vi "Main.vi"() -> ()   [LabVIEW 2017]
doc: "Le programme Main est l'IHM principal du programme MonoSelector. Il controle le sélecteur d'onde de la manipe \"FastFlim\". Il acquit le spectre du laser et permet de positioner le sélecteur ainsi que de choisir la bande passante des ondes lumineuse."
uses:
  Devices/Laser/PulsePickerValues.ctl
  Lib IHM Control/MHL Data.ctl
  Lib IHM Control/MHL UI Data.ctl
  Lib IHM Control/MHL UI Ref.ctl
  Lib IHM Control/Front Panel Status.ctl
  Fonction de transfert/Convertion.ctl
  Lib QMH/MessageQueues.lvlib
  Lib Notifier/Notifier.lvlib
  Lib IHM Control/IHM Control.lvlib
  Lib Log/Logging.lvlib
panel:
  in  "Pulse Picker Set":T1 items=["80"=80, "40"=40, "20"=20, "10"=10, ""=0]
  out "Laser Connection":bool
  in  "LaserON":bool
  out "Power":dbl
  in  "LaserOFF":bool
  out "Pulse Picker":dbl
  in  "Power Set (%)":u8 max=100
  in  "Abort":bool
  in  "Integration (ms)":i32=100
  in  "Stop":bool
  in  "View":bool
  in  "Dlambda +":bool
  in  "Step (mm)":dbl=0.1
  out "lambda":dbl
  in  "Dlambda -":bool
  out "Position (mm)":dbl
  in  "Target (nm)":dbl=480.0
  out "Mono Selector Status":string
  out "Spectrer":cluster{"X":dbl, "Y":dbl}[](graph)
  # "Spectrometer"
  # "Lambda Select"
  # "Laser"
  # "Slite Wide"
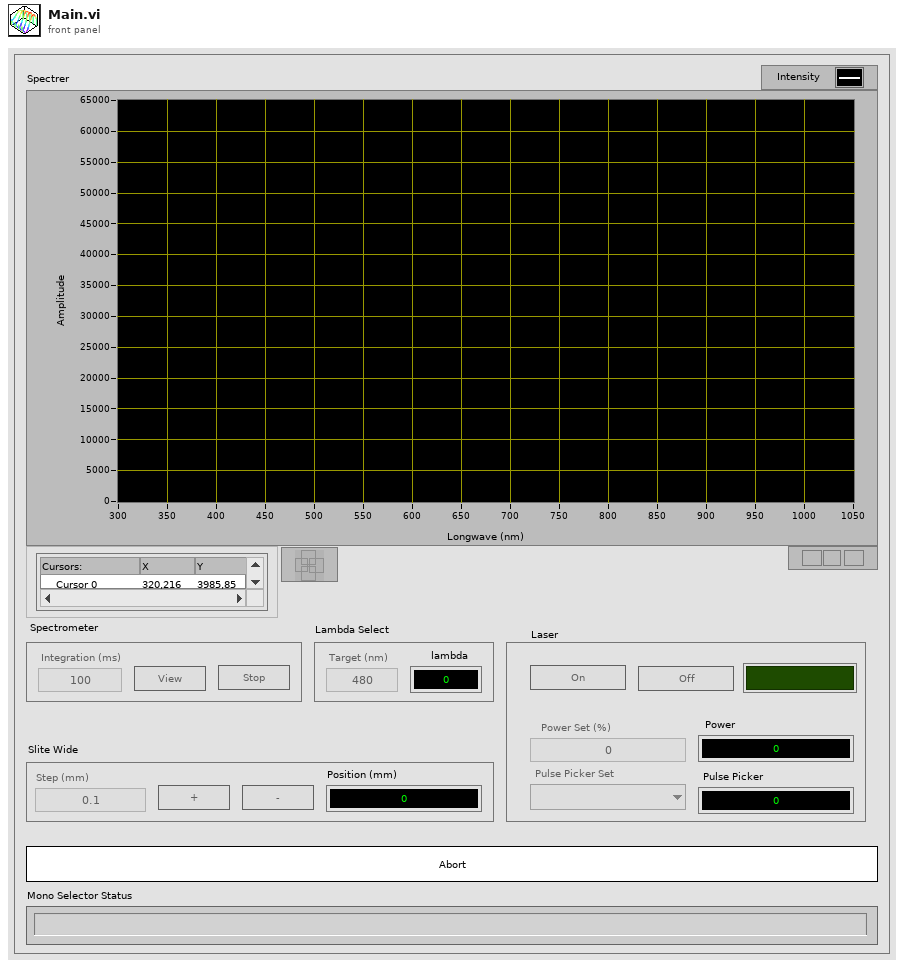
[diagram p1: front panel]
types:
  T1 = typedef "PulsePickerValues.ctl" = u16
  T2 = typedef "MHL Data.ctl" = cluster{"IHM Data":T3, "MHL ref":T4, "Front Panel status":T5}
  T3 = typedef "MHL UI Data.ctl" = cluster{"Integration":i32, "Target Lambda":dbl, "Lambda":dbl, "Step":dbl, "Status Mono":string, "Specter":cluster{"X":dbl, "Y":dbl}[], "Delta Lambda":dbl, "Laser":bool, "Laser Power":dbl, "Pulse Picker Rep. Rate":dbl}
  T4 = typedef "IHM Control.lvlib/MHL UI Ref.ctl" = cluster{"Dlambda-":refnum<vi>, "Abort":refnum<vi>, "Dlambda +":refnum<vi>, "Stop":refnum<vi>, "View":refnum<vi>, "Integration":refnum<vi>, "Target ":refnum<vi>, "Step ":refnum<vi>, "Laser Connection":refnum<vi>, "Power":refnum<vi>, "LaserON":refnum<vi>, "LaserOFF":refnum<vi>, "Pulse Picker Set":refnum<vi>}
  T5 = typedef "IHM Control.lvlib/Front Panel Status.ctl" = enum16{"Initialisation", "Enable Slit", "Enable Positionner", "Enable Spectrometer", "Enable Laser", "Disable Slit", "Disable Positionner", "Disable Spectrometer", "Disable Laser"}
  T6 = typedef "MessageQueues.lvlib/AllMessageQueue Cluster.ctl" = cluster{"MHL":refnum<queue>, "Manager":refnum<queue>, "Recipe":refnum<queue>, "Slit":refnum<queue>, "Positioner":refnum<queue>, "Laser":refnum<queue>, "Spectrometer":refnum<queue>, "Slit Controller":refnum<queue>, "Positioner Controller":refnum<queue>, "Spectrometer Controller":refnum<queue>, "Laser Controller":refnum<queue>}
  T7 = typedef "Notifier.lvlib/Notifier.ctl" = cluster{"Slit Handshake":refnum<notifier>, "Slit Ctrl Exit":refnum<notifier>, "Slit Exit":refnum<notifier>, "Pos. Hanshake":refnum<notifier>, "Pos. Ctrl Exit":refnum<notifier>, "Pos. Exit":refnum<notifier>, "Spectro. Hanshake":refnum<notifier>, "Spectro. Ctrl Exit":refnum<notifier>, "Spectro. Exit":refnum<notifier>, "Laser Handshake":refnum<notifier>, "Laser Ctrl Exit":refnum<notifier>, "Laser Exit":refnum<notifier>}
  T8 = typedef "Convertion.ctl" = enum16{"LongW to Pos.", "Pos. To longW"}
  T9 = enum32{"Invalid", "Standard", "Closed", "Hidden", "Minimized", "Maximized"}
  T10 = enum16{"open", "replace", "create", "open or create", "replace or create", "replace or create with confirmation"}
  T11 = cluster{"état":bool, "code":i32, "source":string}
  T12 = enum32{"invalid app kind", "Development System", "Run Time System", "Student Edition", "Embedded LabVIEW", "Evaluation", "Custom"}
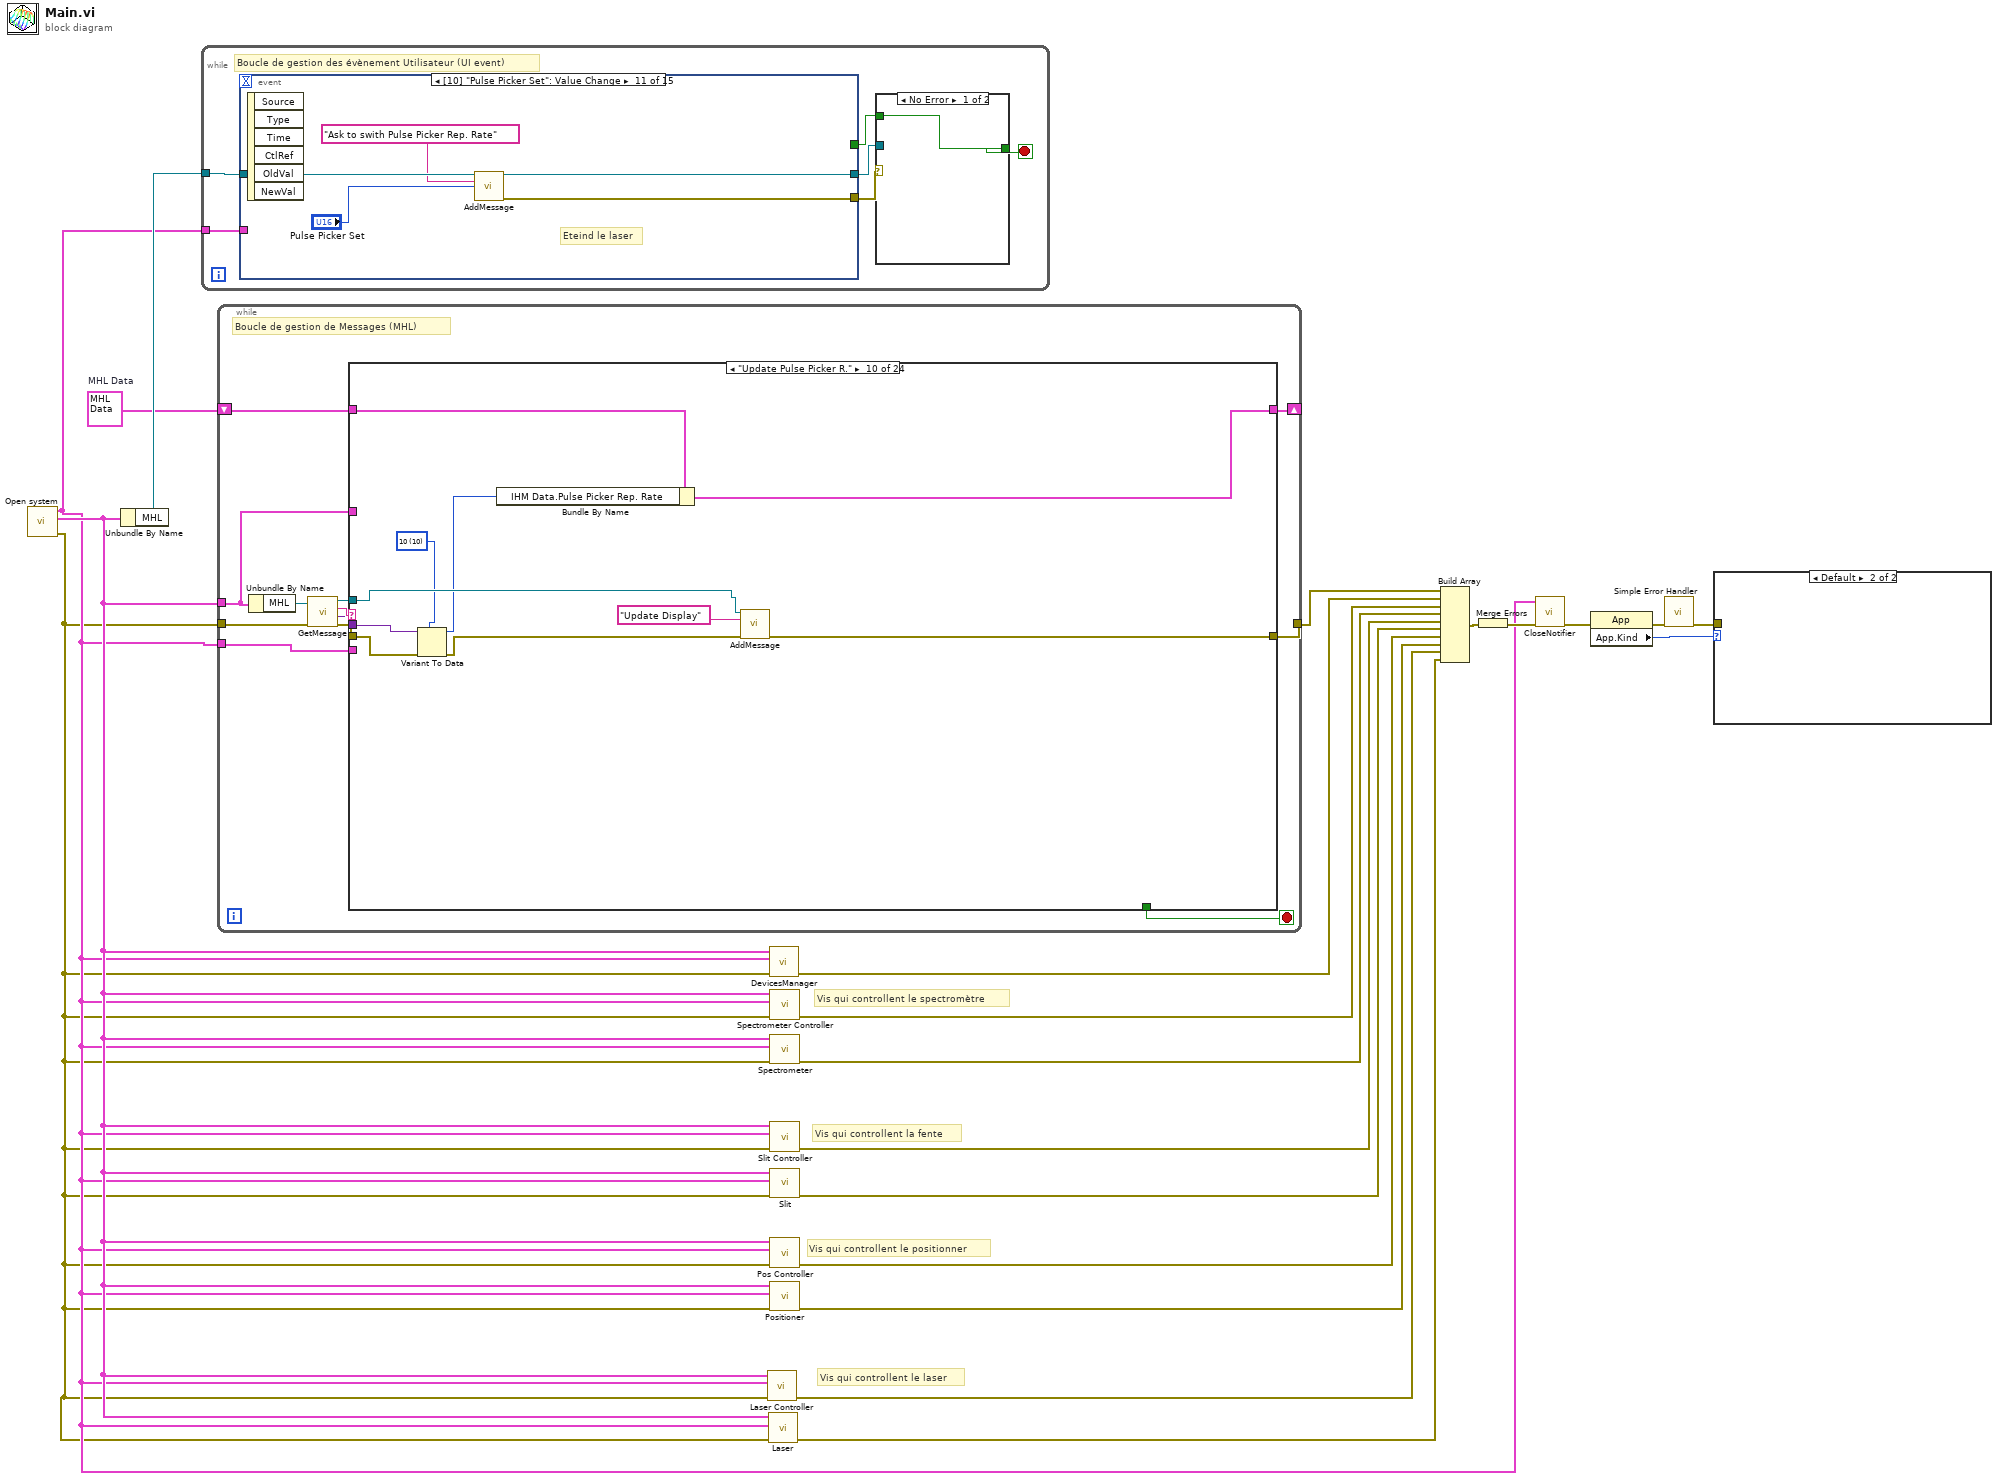
[diagram p0: block diagram]
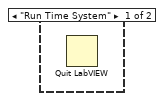
[diagram p2: hidden frame]
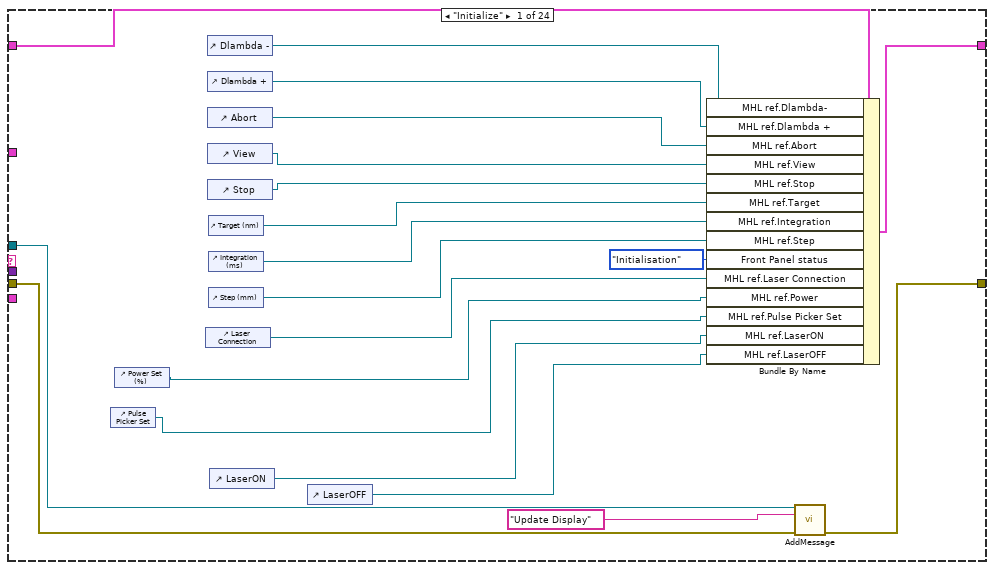
[diagram p3: hidden frame]
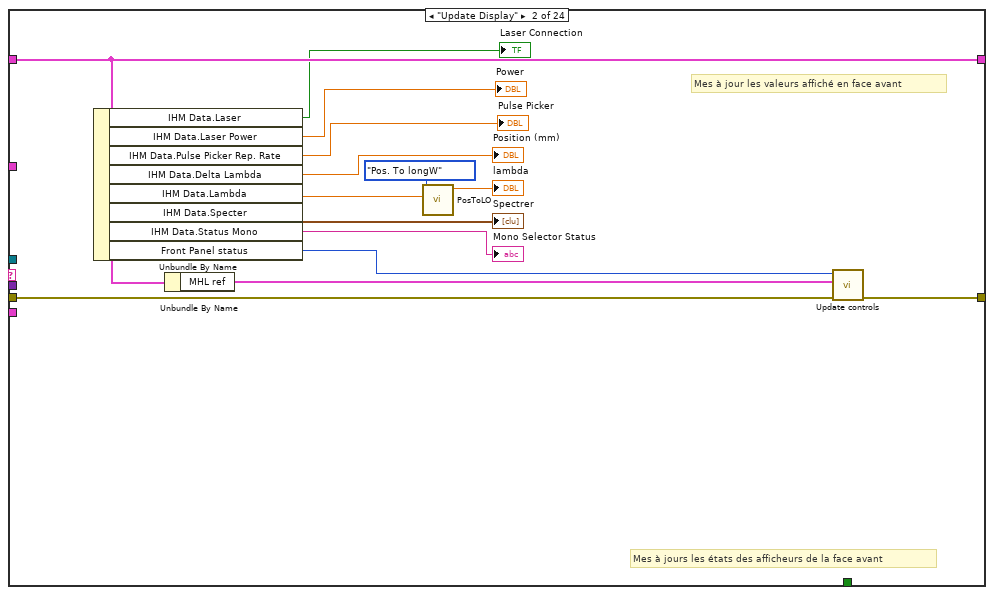
[diagram p4: hidden frame]
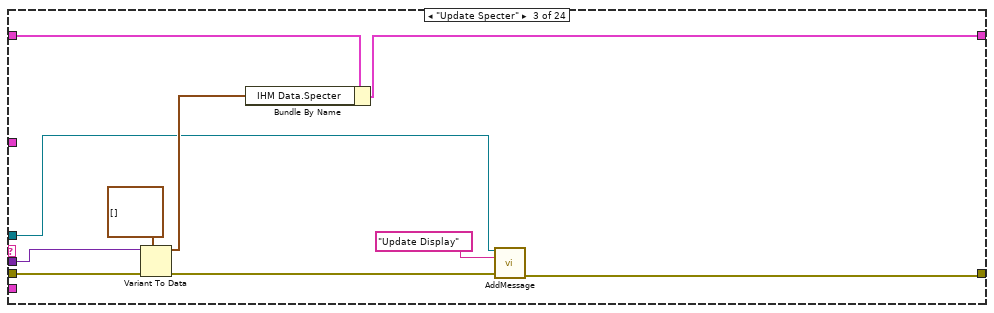
[diagram p5: hidden frame]
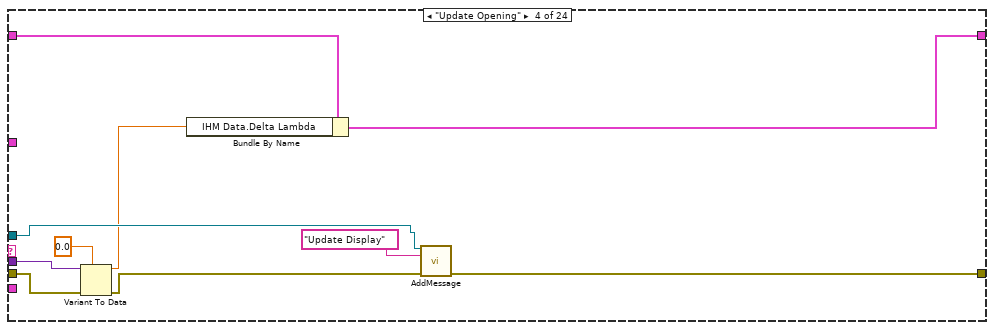
[diagram p6: hidden frame]
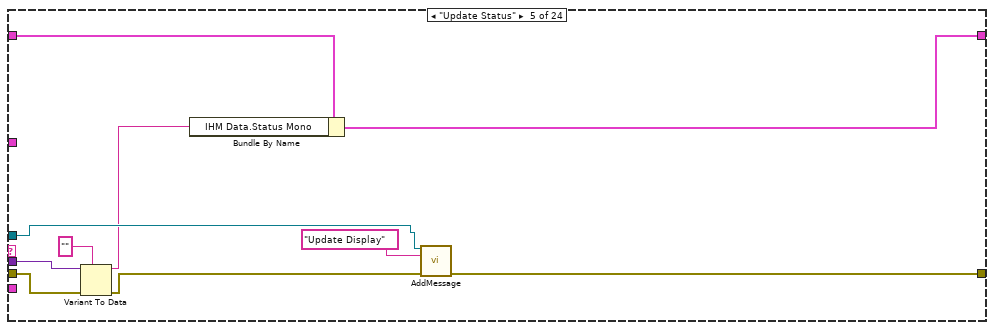
[diagram p7: hidden frame]
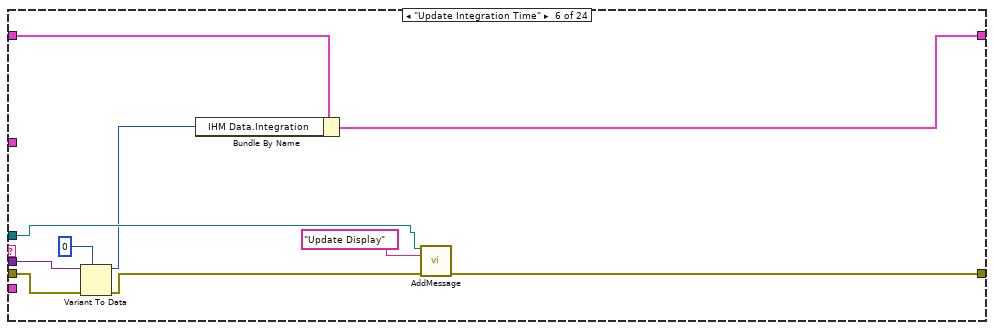
[diagram p8: hidden frame]
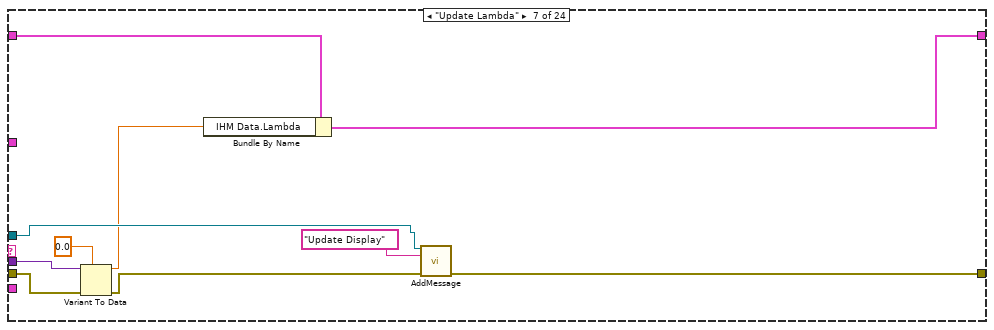
[diagram p9: hidden frame]
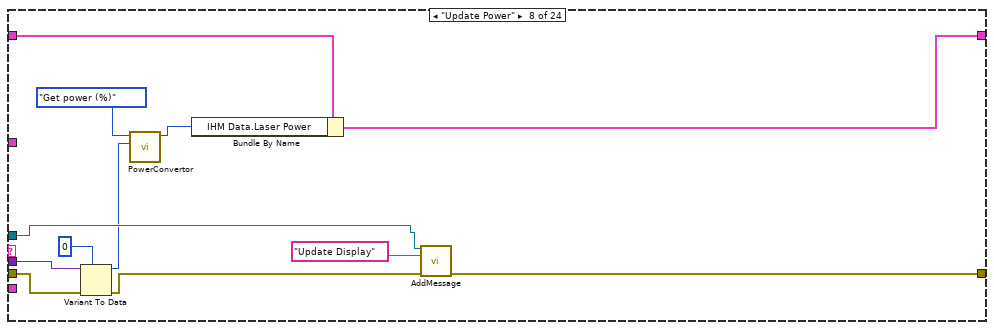
[diagram p10: hidden frame]
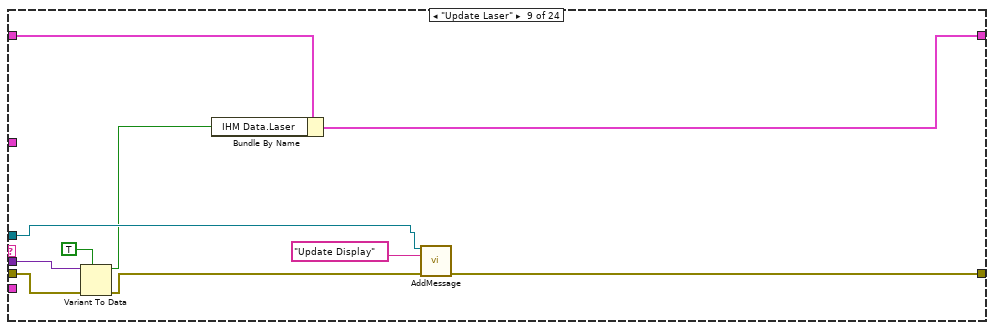
[diagram p11: hidden frame]
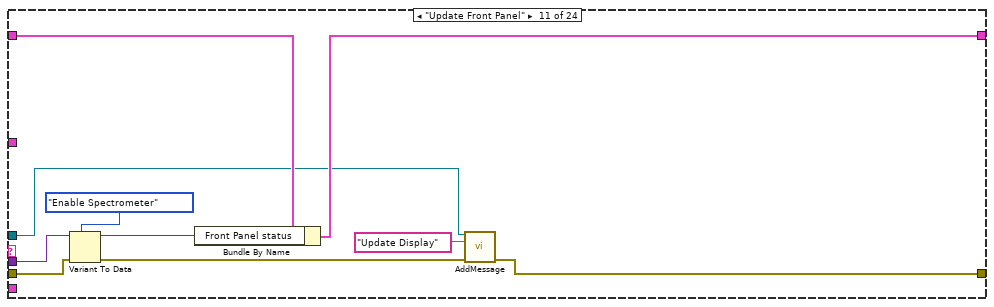
[diagram p12: hidden frame]
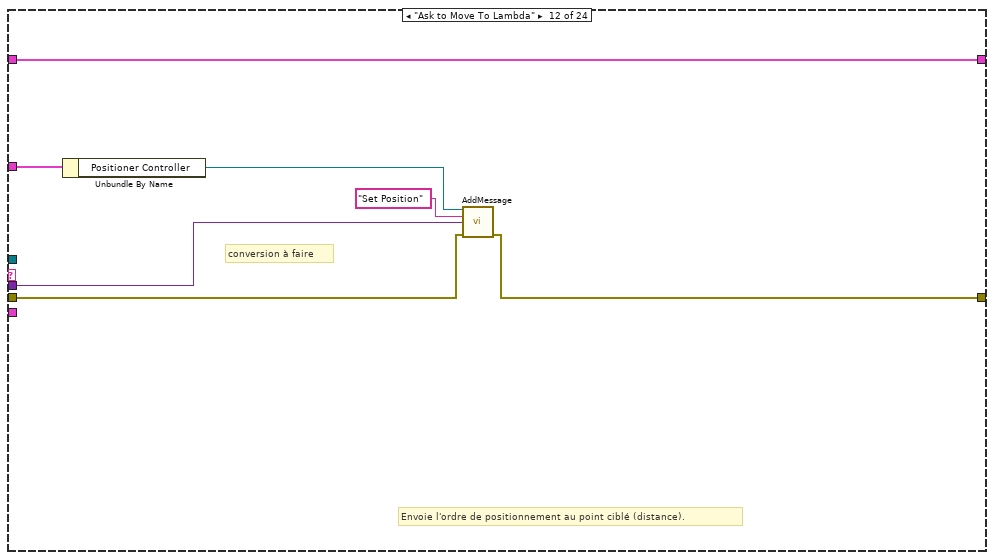
[diagram p13: hidden frame]
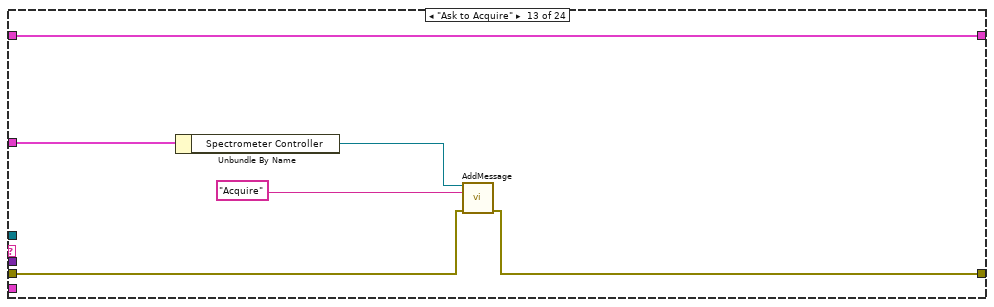
[diagram p14: hidden frame]
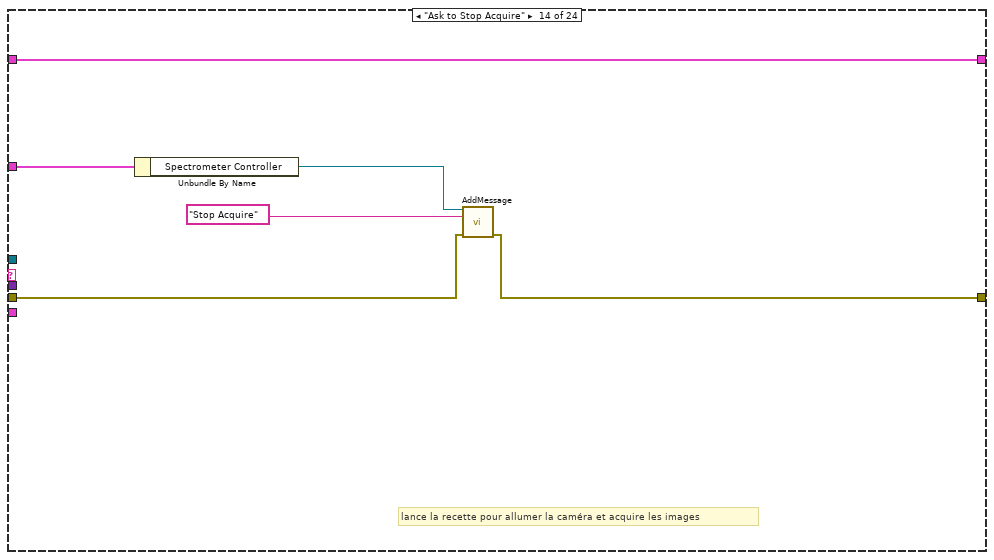
[diagram p15: hidden frame]
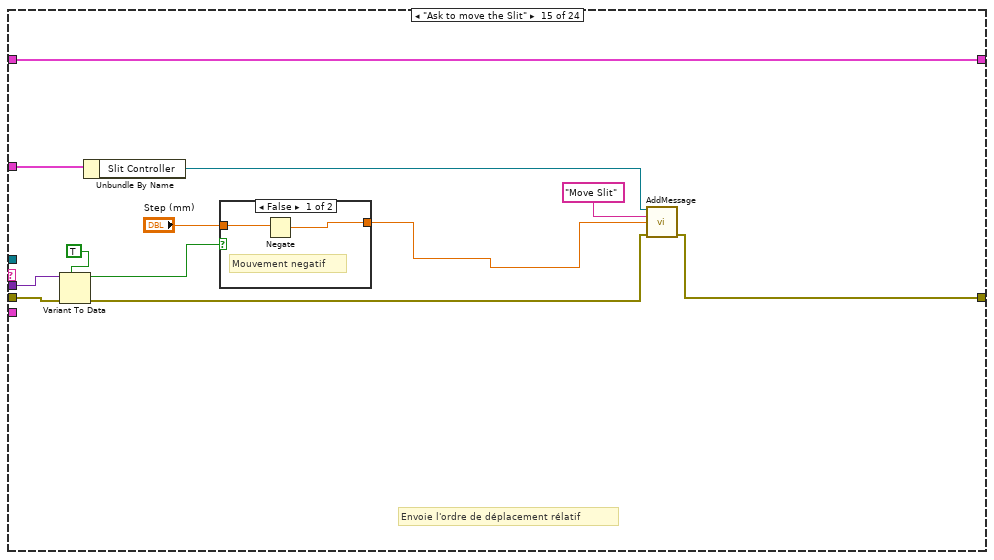
[diagram p16: hidden frame]
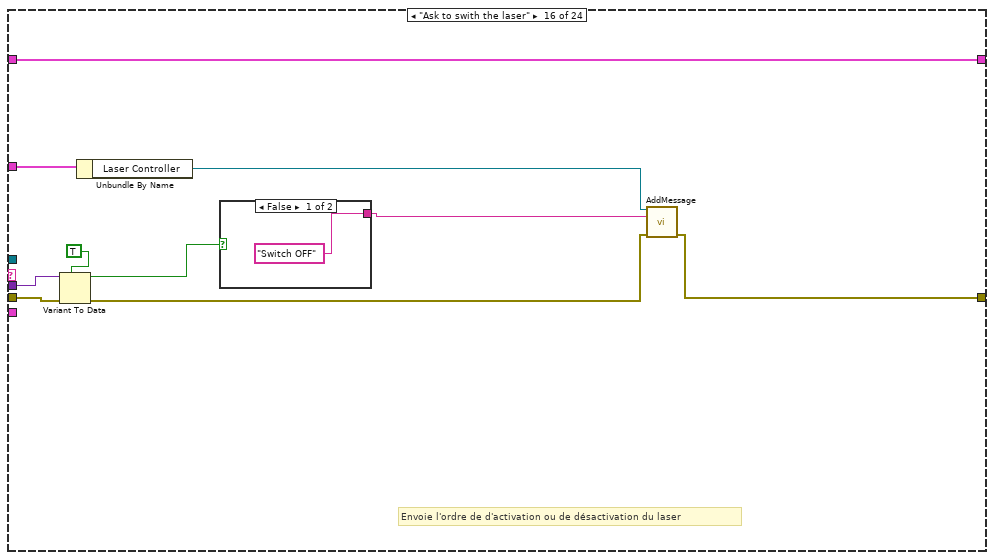
[diagram p18: hidden frame]
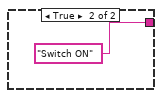
[diagram p19: hidden frame]
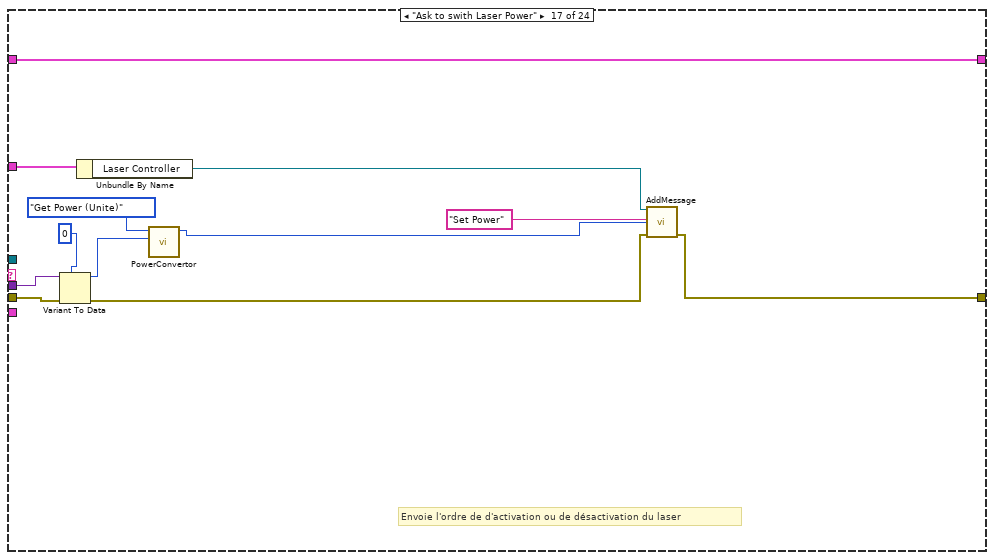
[diagram p20: hidden frame]
diagram:
  w14 = T2 {"IHM Data"={"Integration"=0, "Target Lambda"=0.0, "Lambda"=20.0, "Step"=0.0, "Status Mono"="", "Specter"=[], "Delta Lambda"=0.0, "Laser"=FALSE, "Laser Power"=0.0, "Pulse Picker Rep. Rate"=0.0}, "MHL ref"={"Dlambda-"=refnum, "Abort"=refnum, "Dlambda +"=refnum, "Stop"=refnum, "View"=refnum, "Integration"=refnum, "Target "=refnum, "Step "=refnum, "Laser Connection"=refnum, "Power"=refnum, "LaserON"=refnum, "LaserOFF"=refnum, "Pulse Picker Set"=refnum}, "Front Panel status"=enum."Initialisation"}  # MHL Data
  # "Vis qui controllent le laser"
  # "Vis qui controllent le positionner"
  # "Vis qui controllent la fente"
  # "Vis qui controllent le spectromètre"
  n1 = call "Open system.vi"() -> ("error out"=w3:errorcluster, "All Message Queue Cluster"=w5:T6, "Notifiers"=w4:T7)  [unwired: 8 in, 1 out]
  n2 = Unbundle By Name(w5) -> ("MHL"=w17:refnum<queue>)
  n3 = while {
    tunnel: w17 -> [w27]
    tunnel: w4 -> [w22]
    stop <- w24 stop-if-true
    # "Boucle de gestion des évènement Utilisateur (UI event)"
    n4 = event shown="[10] \"Pulse Picker Set\": Value Change" {
      selector: _ -> [_ _ _ _ _ _ _ _ _ _ _ _ _ _ _]
      dyn-events: _ -> [_ _ _ _ _ _ _ _ _ _ _ _ _ _ _]
      timeout: _ -> [_ _ _ _ _ _ _ _ _ _ _ _ _ _ _]
      tunnel: w27 -> [_ w33 w43 w47 w84 w89 w93 w98 w103 w108 w113 w118 w123 w127 w132]
      tunnel: [_ w34 w40 w45 w81 w86 w90 w95 w100 w105 w110 w115 w120 w124 w130] -> w26
      tunnel: [_ TRUE ("Message Priority ?") _ w44 w82 _ _ _ _ _ _ _ _ _ _] -> w25
      tunnel: [_ w35 w41 w46 w83 w87 w91 w96 w101 w106 w111 w116 w121 w125 w131] -> w23
      tunnel: w22 -> [_ _ _ _ _ _ _ _ _ _ _ _ _ _ _]
      event Timeout {
        n5 = event-data() -> ()  [unwired: 1 in, 2 out]
      }
      event Application Instance Close {
        n6 = event-data() -> ()  [unwired: 1 in, 1 out]
        n7 = call "AddMessage.vi"("Message queue"=w33, "Message"="Initiate Stop") -> ("Dup Message queue"=w35:refnum<queue>, "error out"=w34:errorcluster)  [unwired: 12 in]
      }
      event "Target (nm)": Value Change {
        # "Demande un déplacement vers la lambda demandé"
        n8 = event-data() -> ()  [unwired: 1 in, 1 out]
        n9 = call "PosToLO.vi"("Convertion"=Convertion."LongW to Pos.", "a"="Target (nm)") -> ("P(a)"=w37:dbl)  [unwired: 8 in]
        n10 = call "AddMessage.vi"("Message queue"=w43, "Message"="Ask to Move To Lambda", "Data"=w37) -> ("Dup Message queue"=w41:refnum<queue>, "error out"=w40:errorcluster)  [unwired: 11 in]
      }
      event Menu Selection (User) {
        n11 = event-data() -> ("ItemTag"=w48:string)  [unwired: 1 in]
        n12 = case shown="\"Laser\"" w48 {
          tunnel: w47 -> [w49 w54 w58 w62 w63 w69 w78]
          tunnel: [w49 w54 w58 w62 w63 w69 w77] -> w46
          tunnel: [_ _ _ _ _ _ w76] -> w45
          tunnel: [_ _ _ _ _ _ TRUE ("Message Priority ?")] -> w44
          frame Default {
          }
          frame "Spectrometer" {
            # "Ouvre la FA du spectro"
            n13 = call <vilib>:"Application Directory.vi"() -> ("Application Directory"=w51:path)
            n14 = Build Path(base path=w51, name or relative path="Devices\\Spectrometer\\Spectrometer.vi") -> (appended path=w50:path)
            n15 = Open VI Reference(vi path=w50) -> (vi reference=w53:refnum<vi>)  [unwired: 5 in, 1 out]
            n16 = invoke class="VI" method="FP.Open"(reference=w53) -> ()  [unwired: 4 in, 5 out]
          }
          frame "Manager" {
            # "Ouvre la FA du spectro"
            n17 = vi-ref "DevicesManager.vi"() -> (w55:refnum<vi>)
            n18 = invoke class="VI" method="FP.Open"(reference=w55, "Activate"=TRUE ("Activate?"), "State"=T9."Standard") -> ()  [unwired: 2 in, 5 out]
          }
          frame "Slit" {
            # "Ouvre la FA du Slit"
            n19 = vi-ref "Slit.vi"() -> (w61:refnum<vi>)
            n20 = invoke class="VI Interface Type 0" method="FP.Open"(reference=w61, "Activate"=TRUE ("Activate?"), "State"=T9."Standard") -> ()  [unwired: 2 in, 5 out]
          }
          frame "Selector" {
            # "Ouvre la FA du moteur Ox"
            n21 = call <vilib>:"Application Directory.vi"() -> ("Application Directory"=w65:path)
            n22 = Build Path(base path=w65, name or relative path="Devices\\Positioner\\Positioner.vi") -> (appended path=w66:path)
            n23 = Open VI Reference(vi path=w66) -> (vi reference=w68:refnum<vi>, error out=w67:errorcluster)  [unwired: 5 in]
            n24 = invoke class="VI" method="FP.Open"(reference=w68, error in=w67) -> ()  [unwired: 3 in, 5 out]
          }
          frame "Laser" {
            # "Ouvre la FA du moteur Ox"
            n25 = call <vilib>:"Application Directory.vi"() -> ("Application Directory"=w71:path)
            n26 = Build Path(base path=w71, name or relative path="Devices\\Laser\\Laser.vi") -> (appended path=w72:path)
            n27 = Open VI Reference(vi path=w72) -> (vi reference=w74:refnum<vi>, error out=w73:errorcluster)  [unwired: 5 in]
            n28 = invoke class="VI" method="FP.Open"(reference=w74, error in=w73) -> ()  [unwired: 3 in, 5 out]
          }
          frame "Quit" {
            n29 = call "AddMessage.vi"("Message queue"=w78, "Message"="Initiate Stop") -> ("Dup Message queue"=w77:refnum<queue>, "error out"=w76:errorcluster)  [unwired: 12 in]
          }
        }
      }
      event Panel Close? {
        w82 = TRUE ("Message Priority ?")
        n30 = event-data() -> ()  [unwired: 1 in, 4 out]
        n31 = call "AddMessage.vi"("Message queue"=w84, "Message"="Initiate Stop") -> ("Dup Message queue"=w83:refnum<queue>, "error out"=w81:errorcluster)  [unwired: 12 in]
        n32 = Wait (ms)(milliseconds to wait=u32 500) -> ()  [unwired: 1 out]
        n33 = event-data("Discard?"=w82) -> ()  [unwired: 1 in, 1 out]
      }
      event "View": Value Change {
        # "demande le déplacement du moteur à vers le position mémorisée dans Reg X"
        n34 = event-data() -> ()  [unwired: 1 in, 6 out]
        n35 = call "AddMessage.vi"("Message queue"=w89, "Message"="Ask to Acquire") -> ("Dup Message queue"=w87:refnum<queue>, "error out"=w86:errorcluster)  [unwired: 12 in]
      }
      event "Stop": Value Change {
        # "demande le déplacement du moteur à vers le position mémorisée dans Reg X"
        n36 = event-data() -> ()  [unwired: 1 in, 1 out]
        n37 = call "AddMessage.vi"("Message queue"=w93, "Message"="Ask to Stop Acquire") -> ("Dup Message queue"=w91:refnum<queue>, "error out"=w90:errorcluster)  [unwired: 12 in]
      }
      event "Dlambda +": Value Change {
        # "demande le déplacement du moteur à vers le position mémorisée dans Reg X"
        n38 = event-data() -> ()  [unwired: 1 in, 6 out]
        n39 = call "AddMessage.vi"("Message queue"=w98, "Message"="Ask to move the Slit", "Data"=TRUE ("Dlambda +")) -> ("Dup Message queue"=w96:refnum<queue>, "error out"=w95:errorcluster)  [unwired: 11 in]
      }
      event "LaserON": Value Change {
        # "Allume le laser"
        n40 = event-data() -> ()  [unwired: 1 in, 6 out]
        n41 = call "AddMessage.vi"("Message queue"=w103, "Message"="Ask to swith the laser", "Data"=TRUE ("Dlambda +")) -> ("Dup Message queue"=w101:refnum<queue>, "error out"=w100:errorcluster)  [unwired: 11 in]
      }
      event "LaserOFF": Value Change {
        # "Eteind le laser"
        n42 = event-data() -> ()  [unwired: 1 in, 6 out]
        n43 = call "AddMessage.vi"("Message queue"=w108, "Message"="Ask to swith the laser", "Data"=FALSE ("Dlambda +")) -> ("Dup Message queue"=w106:refnum<queue>, "error out"=w105:errorcluster)  [unwired: 11 in]
      }
      event Value Change {
        # "Eteind le laser"
        n44 = event-data() -> ()  [unwired: 1 in, 6 out]
        n45 = call "AddMessage.vi"("Message queue"=w113, "Message"="Ask to swith Pulse Picker Rep. Rate", "Data"="Pulse Picker Set") -> ("Dup Message queue"=w111:refnum<queue>, "error out"=w110:errorcluster)  [unwired: 11 in]
      }
      event "Power Set (%)": Value Change {
        # "Eteind le laser"
        n46 = event-data() -> ()  [unwired: 1 in, 6 out]
        n47 = call "AddMessage.vi"("Message queue"=w118, "Message"="Ask to swith Laser Power", "Data"="Power Set (%)") -> ("Dup Message queue"=w116:refnum<queue>, "error out"=w115:errorcluster)  [unwired: 11 in]
      }
      event "Dlambda -": Value Change {
        # "demande le déplacement du moteur à vers le position mémorisée dans Reg X"
        n48 = event-data() -> ()  [unwired: 1 in, 6 out]
        n49 = call "AddMessage.vi"("Message queue"=w123, "Message"="Ask to move the Slit", "Data"=FALSE ("Dlambda +")) -> ("Dup Message queue"=w121:refnum<queue>, "error out"=w120:errorcluster)  [unwired: 11 in]
      }
      event "Abort": Value Change {
        # "demande d'annulation d'action des appareils"
        n50 = event-data() -> ()  [unwired: 1 in, 6 out]
        n51 = call "AddMessage.vi"("Message queue"=w127, "Message"="Ask to Abort") -> ("Dup Message queue"=w125:refnum<queue>, "error out"=w124:errorcluster)  [unwired: 12 in]
      }
      event "Integration (ms)": Value Change {
        n52 = event-data() -> ()  [unwired: 1 in, 1 out]
        n53 = call "AddMessage.vi"("Message queue"=w132, "Message"="Set Integration Time", "Data"="Integration (ms)") -> ("Dup Message queue"=w131:refnum<queue>, "error out"=w130:errorcluster)  [unwired: 11 in]
      }
    }
    n54 = case shown="No Error" w26 {
      tunnel: [w28 TRUE ("Message Priority ?")] -> w24
      tunnel: w25 -> [w28 _]
      tunnel: w23 -> [_ w30]
      frame No Error {
      }
      frame Error {
        # "une erreur ferme \nla MHL et stop la boucle\névènementielle"
        n55 = call "AddMessage.vi"("Message queue"=w30, "Message"="Exit") -> ()  [unwired: 12 in, 2 out]
      }
    }
  }
  n56 = while {
    tunnel: w4 -> [w142]
    tunnel: w5 -> [w141]
    shift-right: [w133] -> _
    shift-left: w14 -> [w134]
    tunnel: w3 -> [w139]
    tunnel: [w144] -> w7
    stop <- w143 stop-if-true
    # "Boucle de gestion de Messages (MHL)"
    n57 = Unbundle By Name(w141) -> ("MHL"=w140:refnum<queue>)
    n58 = call "GetMessage.vi"("entrée d'erreur"=w139, "Message queue"=w140) -> ("sortie d'erreur"=w138:errorcluster, "Data"=w135:variant, "Message"=w136:string, "Dup Message Queue"=w137:refnum<queue>)  [unwired: 6 in]
    n59 = case shown="\"Update Pulse Picker R.\"" w136 {
      tunnel: w141 -> [_ _ _ _ _ _ _ _ _ _ _ w277 w283 w289 w301 w314 w328 w335 w344 w355 _ _ _ w407]
      tunnel: w137 -> [w160 _ w180 w196 w206 w216 w226 w238 w248 w258 w262 _ _ _ _ _ _ _ _ _ w360 _ w390 _]
      tunnel: w138 -> [w162 w178 w187 w193 w203 w213 w223 w235 w246 w256 w270 w274 w280 w286 w296 w310 w324 w330 w340 w352 w369 w386 w389 w395]
      tunnel: [w161 w177 w181 w197 w207 w217 w227 w239 w249 w259 w263 w273 w279 w285 w298 w312 w326 w333 w345 w346 w361 w386 w388 w399] -> w144
      tunnel: [_ _ _ _ _ _ _ _ _ _ _ _ _ _ _ _ _ _ _ _ _ _ TRUE _] -> w143
      tunnel: w142 -> [_ _ _ _ _ _ _ _ _ _ _ _ _ _ _ _ _ _ _ _ _ _ _ _]
      tunnel: w135 -> [_ _ w186 w195 w205 w215 w225 w237 w247 w257 w269 w271 _ _ w293 w307 w322 w329 w338 _ w368 _ _ _]
      tunnel: w134 -> [w164 w175 w188 w191 w201 w211 w221 w233 w244 w254 w267 w272 w278 w284 w297 w311 w325 w332 w341 w353 w359 w384 w387 w406]
      tunnel: [w163 w175 w179 w190 w200 w210 w220 w232 w243 w253 w265 w272 w278 w284 w297 w311 w325 w332 w341 w353 w356 w384 w387 w406] -> w133
      frame "Initialize" {
        n60 = control-ref of="Pulse Picker Set"() -> (w145:refnum<vi>)
        n61 = control-ref of="Power Set (%)"() -> (w146:refnum<vi>)
        n62 = control-ref of="Laser Connection"() -> (w149:refnum<vi>)
        n63 = control-ref of="Dlambda -"() -> (w158:refnum<vi>)
        n64 = control-ref of="Dlambda +"() -> (w157:refnum<vi>)
        n65 = control-ref of="Abort"() -> (w156:refnum<vi>)
        n66 = control-ref of="View"() -> (w155:refnum<vi>)
        n67 = control-ref of="Stop"() -> (w154:refnum<vi>)
        n68 = control-ref of="Target (nm)"() -> (w153:refnum<vi>)
        n69 = control-ref of="Integration (ms)"() -> (w152:refnum<vi>)
        n70 = control-ref of="Step (mm)"() -> (w151:refnum<vi>)
        n71 = control-ref of="LaserON"() -> (w148:refnum<vi>)
        n72 = control-ref of="LaserOFF"() -> (w147:refnum<vi>)
        n73 = Bundle By Name(cluster=w164, "MHL ref.Dlambda-"=w158, "MHL ref.Dlambda +"=w157, "MHL ref.Abort"=w156, "MHL ref.View"=w155, "MHL ref.Stop"=w154, "MHL ref.Target"=w153, "MHL ref.Integration"=w152, "MHL ref.Step"=w151, "Front Panel status"=Front_Panel_Status."Initialisation", "MHL ref.Laser Connection"=w149, "MHL ref.Power"=w146, "MHL ref.Pulse Picker Set"=w145, "MHL ref.LaserON"=w148, "MHL ref.LaserOFF"=w147) -> (w163:T2)
        n74 = call "AddMessage.vi"("Message queue"=w160, "Message"="Update Display", "entrée d'erreur (pas d'erreur)"=w162) -> ("error out"=w161:errorcluster)  [unwired: 11 in, 1 out]
      }
      frame "Update Display" {
        # "Mes à jours les états des afficheurs de la face avant"
        # "Mes à jour les valeurs affiché en face avant"
        n75 = Unbundle By Name(w175) -> ("IHM Data.Laser"=→"Laser Connection":bool, "IHM Data.Laser Power"=→"Power":dbl, "IHM Data.Pulse Picker Rep. Rate"=→"Pulse Picker":dbl, "IHM Data.Delta Lambda"=→"Position (mm)":dbl, "IHM Data.Lambda"=w170:dbl, "IHM Data.Specter"=→"Spectrer":cluster{"X":dbl, "Y":dbl}[], "IHM Data.Status Mono"=→"Mono Selector Status":string, "Front Panel status"=w174:T5)
        n76 = Unbundle By Name(w175) -> ("MHL ref"=w176:T4)
        n77 = call "PosToLO.vi"("Convertion"=Convertion."Pos. To longW", "a"=w170) -> ("P(a)"=→"lambda":dbl)  [unwired: 8 in]
        n78 = call "Update controls.vi"("error in (no error)"=w178, "IHM Data refnum"=w176, "Front Panel status"=w174) -> ("error out"=w177:errorcluster)  [unwired: 8 in]
      }
      frame "Update Specter" {
        n79 = Variant To Data(error in=w187, type=cluster{"X":dbl, "Y":dbl}[] [] ("IHM Data.Specter"), Variant=w186) -> (data=w184:cluster{"X":dbl, "Y":dbl}[], error out=w182:errorcluster)
        n80 = Bundle By Name(cluster=w188, "IHM Data.Specter"=w184) -> (w179:T2)
        n81 = call "AddMessage.vi"("Message queue"=w180, "Message"="Update Display", "entrée d'erreur (pas d'erreur)"=w182) -> ("error out"=w181:errorcluster)  [unwired: 11 in, 1 out]
      }
      frame "Update Opening" {
        n82 = Variant To Data(error in=w193, type=0.0, Variant=w195) -> (data=w189:dbl, error out=w192:errorcluster)
        n83 = Bundle By Name(cluster=w191, "IHM Data.Delta Lambda"=w189) -> (w190:T2)
        n84 = call "AddMessage.vi"("Message queue"=w196, "Message"="Update Display", "entrée d'erreur (pas d'erreur)"=w192) -> ("error out"=w197:errorcluster)  [unwired: 11 in, 1 out]
      }
      frame "Update Status" {
        n85 = Variant To Data(error in=w203, type="", Variant=w205) -> (data=w199:string, error out=w202:errorcluster)
        n86 = Bundle By Name(cluster=w201, "IHM Data.Status Mono"=w199) -> (w200:T2)
        n87 = call "AddMessage.vi"("Message queue"=w206, "Message"="Update Display", "entrée d'erreur (pas d'erreur)"=w202) -> ("error out"=w207:errorcluster)  [unwired: 11 in, 1 out]
      }
      frame "Update Integration Time" {
        n88 = Variant To Data(error in=w213, type=0, Variant=w215) -> (data=w209:i32, error out=w212:errorcluster)
        n89 = Bundle By Name(cluster=w211, "IHM Data.Integration"=w209) -> (w210:T2)
        n90 = call "AddMessage.vi"("Message queue"=w216, "Message"="Update Display", "entrée d'erreur (pas d'erreur)"=w212) -> ("error out"=w217:errorcluster)  [unwired: 11 in, 1 out]
      }
      frame "Update Lambda" {
        n91 = Variant To Data(error in=w223, type=0.0, Variant=w225) -> (data=w219:dbl, error out=w222:errorcluster)
        n92 = Bundle By Name(cluster=w221, "IHM Data.Lambda"=w219) -> (w220:T2)
        n93 = call "AddMessage.vi"("Message queue"=w226, "Message"="Update Display", "entrée d'erreur (pas d'erreur)"=w222) -> ("error out"=w227:errorcluster)  [unwired: 11 in, 1 out]
      }
      frame "Update Power" {
        n94 = Variant To Data(error in=w235, type=u16 0, Variant=w237) -> (data=w231:u16, error out=w234:errorcluster)
        n95 = call "PowerConvertor.vi"("Power In"=w231, "Action"=enum16{"Get power (%)", "Get Power (Unite)"}."Get power (%)") -> ("Power Out"=w230:u16)  [unwired: 9 in]
        n96 = Bundle By Name(cluster=w233, "IHM Data.Laser Power"=w230) -> (w232:T2)
        n97 = call "AddMessage.vi"("Message queue"=w238, "Message"="Update Display", "entrée d'erreur (pas d'erreur)"=w234) -> ("error out"=w239:errorcluster)  [unwired: 11 in, 1 out]
      }
      frame "Update Laser" {
        n98 = Variant To Data(error in=w246, type=TRUE, Variant=w247) -> (data=w241:bool, error out=w245:errorcluster)
        n99 = Bundle By Name(cluster=w244, "IHM Data.Laser"=w241) -> (w243:T2)
        n100 = call "AddMessage.vi"("Message queue"=w248, "Message"="Update Display", "entrée d'erreur (pas d'erreur)"=w245) -> ("error out"=w249:errorcluster)  [unwired: 11 in, 1 out]
      }
      frame "Update Pulse Picker R." {
        w251 = T1 10 items=["80"=80, "40"=40, "20"=20, "10"=10, ""=0] ("Pulse Picker Set")
        n101 = Variant To Data(error in=w256, type=w251, Variant=w257) -> (data=w252:T1, error out=w255:errorcluster)
        n102 = Bundle By Name(cluster=w254, "IHM Data.Pulse Picker Rep. Rate"=w252) -> (w253:T2)
        n103 = call "AddMessage.vi"("Message queue"=w258, "Message"="Update Display", "entrée d'erreur (pas d'erreur)"=w255) -> ("error out"=w259:errorcluster)  [unwired: 11 in, 1 out]
      }
      frame "Update Front Panel" {
        n104 = Variant To Data(error in=w270, type=Front_Panel_Status."Enable Spectrometer" ("Front Panel status"), Variant=w269) -> (data=w266:T5, error out=w264:errorcluster)
        n105 = Bundle By Name(cluster=w267, "Front Panel status"=w266) -> (w265:T2)
        n106 = call "AddMessage.vi"("Message queue"=w262, "Message"="Update Display", "entrée d'erreur (pas d'erreur)"=w264) -> ("error out"=w263:errorcluster)  [unwired: 11 in, 1 out]
      }
      frame "Ask to Move To Lambda" {
        # "conversion à faire"
        # "Envoie l'ordre de positionnement au point ciblé (distance)."
        n107 = Unbundle By Name(w277) -> ("Positioner Controller"=w276:refnum<queue>)
        n108 = call "AddMessage.vi"("Message queue"=w276, "Message"="Set Position", "Data"=w271, "entrée d'erreur (pas d'erreur)"=w274) -> ("error out"=w273:errorcluster)  [unwired: 10 in, 1 out]
      }
      frame "Ask to Acquire" {
        n109 = Unbundle By Name(w283) -> ("Spectrometer Controller"=w282:refnum<queue>)
        n110 = call "AddMessage.vi"("Message queue"=w282, "Message"="Acquire", "entrée d'erreur (pas d'erreur)"=w280) -> ("error out"=w279:errorcluster)  [unwired: 11 in, 1 out]
      }
      frame "Ask to Stop Acquire" {
        # "lance la recette pour allumer la caméra et acquire les images"
        n111 = Unbundle By Name(w289) -> ("Spectrometer Controller"=w288:refnum<queue>)
        n112 = call "AddMessage.vi"("Message queue"=w288, "Message"="Stop Acquire", "entrée d'erreur (pas d'erreur)"=w286) -> ("error out"=w285:errorcluster)  [unwired: 11 in, 1 out]
      }
      frame "Ask to move the Slit" {
        # "Envoie l'ordre de déplacement rélatif"
        n113 = Variant To Data(error in=w296, type=TRUE, Variant=w293) -> (data=w292:bool, error out=w295:errorcluster)
        n114 = Unbundle By Name(w301) -> ("Slit Controller"=w300:refnum<queue>)
        n115 = case shown="False" w292 {
          tunnel: [w303 w304] -> w290
          tunnel: "Step (mm)" -> [w302 w304]
          frame False {
            # "Mouvement negatif"
            n116 = Negate(x=w302) -> (-x=w303:dbl)
          }
          frame True {
            # "Mouvement positif"
          }
        }
        n117 = call "AddMessage.vi"("Message queue"=w300, "Message"="Move Slit", "Data"=w290, "entrée d'erreur (pas d'erreur)"=w295) -> ("error out"=w298:errorcluster)  [unwired: 10 in, 1 out]
      }
      frame "Ask to swith the laser" {
        # "Envoie l'ordre de d'activation ou de désactivation du laser"
        n118 = Variant To Data(error in=w310, type=TRUE, Variant=w307) -> (data=w306:bool, error out=w309:errorcluster)
        n119 = Unbundle By Name(w314) -> ("Laser Controller"=w313:refnum<queue>)
        n120 = case shown="False" w306 {
          tunnel: ["Switch OFF" ("Message") "Switch ON" ("Message")] -> w305
          frame False {
          }
          frame True {
          }
        }
        n121 = call "AddMessage.vi"("Message queue"=w313, "Message"=w305, "entrée d'erreur (pas d'erreur)"=w309) -> ("error out"=w312:errorcluster)  [unwired: 11 in, 1 out]
      }
      frame "Ask to swith Laser Power" {
        # "Envoie l'ordre de d'activation ou de désactivation du laser"
        n122 = Variant To Data(error in=w324, type=u8 0 ("Power Set (%)"), Variant=w322) -> (data=w319:u8, error out=w323:errorcluster)
        n123 = Unbundle By Name(w328) -> ("Laser Controller"=w327:refnum<queue>)
        n124 = call "PowerConvertor.vi"("Power In"=w319, "Action"=enum16{"Get power (%)", "Get Power (Unite)"}."Get Power (Unite)") -> ("Power Out"=w317:u16)  [unwired: 9 in]
        n125 = call "AddMessage.vi"("Message queue"=w327, "Message"="Set Power", "Data"=w317, "entrée d'erreur (pas d'erreur)"=w323) -> ("error out"=w326:errorcluster)  [unwired: 10 in, 1 out]
      }
      frame "Ask to swith Pulse Picker Rep. Rate" {
        # "Envoie l'ordre de changer la frequencce du pulse picker"
        n126 = Unbundle By Name(w335) -> ("Laser Controller"=w334:refnum<queue>)
        n127 = call "AddMessage.vi"("Message queue"=w334, "Message"="Set Pulse Picker", "Data"=w329, "entrée d'erreur (pas d'erreur)"=w330) -> ("error out"=w333:errorcluster)  [unwired: 10 in, 1 out]
      }
      frame "Set Integration Time" {
        # "Met à jour  la registre correspond à la vitesse"
        n128 = Unbundle By Name(w344) -> ("Spectrometer Controller"=w343:refnum<queue>)
        n129 = Variant To Data(error in=w340, type=3 ("Integration (ms)"), Variant=w338) -> (data=w336:i32, error out=w339:errorcluster)
        n130 = Bundle By Name(cluster=w341, "IHM Data.Integration"=w336) -> ()  [unwired: 1 out]
        n131 = call "AddMessage.vi"("Message queue"=w343, "Message"="Set Integration Time", "Data"=w336, "entrée d'erreur (pas d'erreur)"=w339) -> ("error out"=w345:errorcluster)  [unwired: 10 in, 1 out]
      }
      frame "Ask to Abort" {
        w349 = "Abort" ("Message")
        # "Envoie l'ordre d'annulation chaques appareils."
        n132 = Unbundle By Name(w355) -> ("Slit Controller"=w350:refnum<queue>, "Positioner Controller"=w351:refnum<queue>, "Spectrometer Controller"=w354:refnum<queue>)
        n133 = call "AddMessage.vi"("Message queue"=w354, "Message"=w349, "entrée d'erreur (pas d'erreur)"=w352) -> ("error out"=w348:errorcluster)  [unwired: 11 in, 1 out]
        n134 = call "AddMessage.vi"("Message queue"=w351, "Message"=w349, "entrée d'erreur (pas d'erreur)"=w348) -> ("error out"=w347:errorcluster)  [unwired: 11 in, 1 out]
        n135 = call "AddMessage.vi"("Message queue"=w350, "Message"=w349, "entrée d'erreur (pas d'erreur)"=w347) -> ("error out"=w346:errorcluster)  [unwired: 11 in, 1 out]
      }
      frame "Erreur" {
        n136 = Variant To Data(error in=w369, type=T11 {"état"=FALSE, "code"=0, "source"=""} ("sortie d'erreur"), Variant=w368) -> (data=w377:T11, error out=w378:errorcluster)
        n137 = call <vilib>:"Application Directory.vi"() -> ("Application Directory"=w375:path)
        n138 = Merge Errors(w377, w378) -> (w376:errorcluster)
        n139 = Unbundle By Name(w376) -> ("source"=w358:string, "code"=w365:i32)
        n140 = Build Path(base path=w375, name or relative path=path "Error Log.txt") -> (appended path=w374:path)
        n141 = Open/Create/Replace File(file path (use dialog)=w374, operation (0:open)=T10."open or create" ("opération (0 : open)")) -> (refnum out=w367:refnum<file>, error out=w370:errorcluster)  [unwired: 4 in, 1 out]
        n142 = call <vilib>:"Clear Errors.vi"("error in (no error)"=w370) -> ("error out"=w364:errorcluster)  [unwired: 5 in, 1 out]
        n143 = Bundle By Name(cluster=w359, "IHM Data.Status Mono"=w358) -> (w356:T2)
        n144 = call "LogError.vi"("entrée d'erreur"=w364, "Code"=w365, "Source"=w358, "Error log refnum In"=w367) -> ("error out"=w363:errorcluster, "Error log refnum out"=w366:refnum<file>)  [unwired: 6 in]
        n145 = Not A Number/Path/Refnum?(number/path/refnum=w366) -> (NaN/Path/Refnum?=w371:bool)
        n146 = case shown="False" w371 {
          tunnel: w363 -> [w382 w383]
          tunnel: w366 -> [w381 _]
          tunnel: [w380 w383] -> w362
          frame False {
            n147 = Close File(refnum=w381, error in=w382) -> (error out=w380:errorcluster)  [unwired: 1 out]
          }
          frame True {
          }
        }
        n148 = call "AddMessage.vi"("Message queue"=w360, "Message"="Update Display", "entrée d'erreur (pas d'erreur)"=w362) -> ("error out"=w361:errorcluster)  [unwired: 11 in, 1 out]
      }
      frame Default {
        n149 = One Button Dialog(message="Warning : Message erroné ou erreur dans le MHL") -> ()  [unwired: 1 in, 1 out]
      }
      frame "Quit" {
        # "Libère la pile MHL et stop la boucle"
        n150 = Release Queue(queue=w390, error in (no error)=w389) -> (error out=w388:errorcluster)  [unwired: 1 in, 2 out]
      }
      frame "Initiate Stop" {
        w393 = "Exit" ("Message")
        # "Envoie un message d'arrête à tous les controleur.\nPuis demande d'attendre jusqu'à ce que chaque appareils soit arrêtés"
        n151 = Unbundle By Name(w407) -> ("MHL"=w398:refnum<queue>, "Slit Controller"=w405:refnum<queue>, "Positioner Controller"=w404:refnum<queue>, "Spectrometer Controller"=w403:refnum<queue>, "Manager"=w396:refnum<queue>, "Laser Controller"=w392:refnum<queue>)
        n152 = call "AddMessage.vi"("Message queue"=w404, "Message"=w393, "entrée d'erreur (pas d'erreur)"=w395) -> ("error out"=w401:errorcluster)  [unwired: 11 in, 1 out]
        n153 = call "AddMessage.vi"("Message queue"=w403, "Message"=w393, "entrée d'erreur (pas d'erreur)"=w395) -> ("error out"=w400:errorcluster)  [unwired: 11 in, 1 out]
        n154 = call "AddMessage.vi"("Message queue"=w396, "Message"=w393, "entrée d'erreur (pas d'erreur)"=w395) -> ("error out"=w397:errorcluster)  [unwired: 11 in, 1 out]
        n155 = call "AddMessage.vi"("Message queue"=w405, "Message"=w393, "entrée d'erreur (pas d'erreur)"=w395) -> ("error out"=w402:errorcluster)  [unwired: 11 in, 1 out]
        n156 = call "AddMessage.vi"("Message queue"=w392, "Message"=w393, "entrée d'erreur (pas d'erreur)"=w395) -> ("error out"=w394:errorcluster)  [unwired: 11 in, 1 out]
        n157 = Merge Errors(w402, w401, w400, w397, w394) -> (w399:errorcluster)
        n158 = case shown="No Error" w399 {
          selector: w399 -> [w408 _]
          tunnel: w398 -> [w410 _]
          frame No Error {
            n159 = call "AddMessage.vi"("Message queue"=w410, "Message"="Quit", "entrée d'erreur (pas d'erreur)"=w408) -> ()  [unwired: 11 in, 2 out]
          }
          frame Error {
          }
        }
      }
    }
  }
  n160 = call "Laser Controller.vi"("error in (no error)"=w3, "Notifiers"=w4, "All Message Queue Cluster"=w5) -> ("error out"=w2:errorcluster)  [unwired: 8 in]
  n161 = call "Laser.vi"("error in (no error)"=w3, "Notifiers"=w4, "All Message Queue Cluster"=w5) -> ("error out"=w1:errorcluster)  [unwired: 8 in]
  n162 = call "DevicesManager.vi"("error in (no error)"=w3, "Notifiers"=w4, "All Message Queue Cluster"=w5) -> ("error out"=w6:errorcluster)  [unwired: 8 in]
  n163 = call "Spectrometer Controller.vi"("error in (no error)"=w3, "Notifiers"=w4, "All Message Queue Cluster"=w5) -> ("error out"=w13:errorcluster)  [unwired: 8 in]
  n164 = call "Spectrometer.vi"("error in (no error)"=w3, "Notifiers"=w4, "All Message Queue Cluster"=w5) -> ("error out"=w12:errorcluster)  [unwired: 8 in]
  n165 = call "Slit Controller.vi"("error in (no error)"=w3, "Notifiers"=w4, "All Message Queue Cluster"=w5) -> ("error out"=w11:errorcluster)  [unwired: 8 in]
  n166 = call "Slit.vi"("error in (no error)"=w3, "Notifiers"=w4, "All Message Queue Cluster"=w5) -> ("error out"=w10:errorcluster)  [unwired: 8 in]
  n167 = call "Pos Controller.vi"("error in (no error)"=w3, "Notifiers"=w4, "All Message Queue Cluster"=w5) -> ("error out"=w9:errorcluster)  [unwired: 8 in]
  n168 = call "Positioner.vi"("error in (no error)"=w3, "Notifiers"=w4, "All Message Queue Cluster"=w5) -> ("error out"=w8:errorcluster)  [unwired: 8 in]
  n169 = Build Array(w7, w6, w13, w12, w11, w10, w9, w8, w2, w1) -> (w21:errorcluster[])
  n170 = Merge Errors(w21) -> (w16:errorcluster)
  n171 = call "CloseNotifier.vi"("entrée d'erreur"=w16, "Notifiers"=w4) -> ("error out"=w15:errorcluster)  [unwired: 9 in]
  n172 = property class="App"(error in=w15) -> (error out=w19:errorcluster, "App.Kind"=w20:T12)  [unwired: 1 in, 1 out]
  n173 = call <vilib>:"Simple Error Handler.vi"("error in (no error)"=w19) -> ("error out"=w18:errorcluster)  [unwired: 4 in, 4 out]
  n174 = case shown="Default" w20 {
    tunnel: w18 -> [_ _]
    frame "Run Time System" {
      n175 = Quit LabVIEW() -> ()  [unwired: 1 in]
    }
    frame Default {
    }
  }
